vi "Write Session Handle.vi"(8 "error in (no error)":errorcluster, 10 "hSerial":T1, 11 "Airmar WS in":refnum<class "Airmar WS.lvclass">) -> (0 "error out":errorcluster, 3 "Airmar WS out":refnum<class "Airmar WS.lvclass">)   [LabVIEW 2014, in "Airmar WS.lvclass"]
uses:
  Airmar WS.lvclass
  <userlib>/_Session Fwk/Typedefs/Session Handle.ctl
  <userlib>/_Session Fwk/Session - Root.lvclass
  Airmar WS.lvclass/Airmar WS.ctl
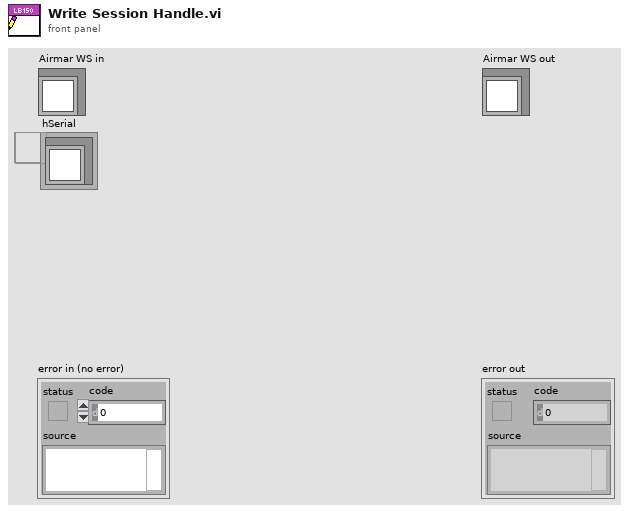
[diagram p1: front panel]
types:
  T1 = typedef "Session - Root.lvclass/Session Handle.ctl" = refnum<data-value>
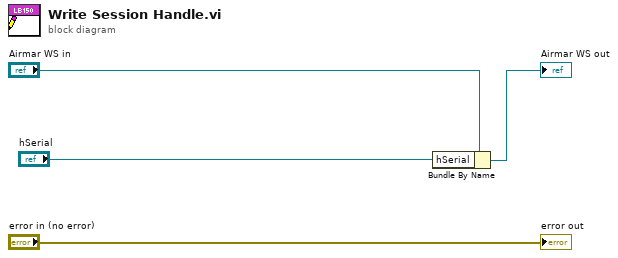
[diagram p0: block diagram]
diagram:
  n1 = Bundle By Name(cluster="Airmar WS in", "hSerial"="hSerial") -> (→"Airmar WS out":refnum<class "Airmar WS.lvclass">)
  "error out" <- "error in (no error)"
